vi "NI5112.start scan.vi"(0 "i ref in":refnum<vi>, 3 "ms timeout (100)":i32=100, 5 "error in (no error)":errorcluster) -> (14 "i ref out":refnum<vi>, 17 "timed out":bool, 19 "error out":errorcluster)   [LabVIEW 2014, in "NI5112.lvlib"]
uses:
  NI5112.lvlib
  <instrlib>/niScope/Controls/niScope trigger source.ctl
  <instrlib>/niScope/Controls/niScope trigger slope.ctl
  <instrlib>/niScope/Controls/niScope trigger coupling.ctl
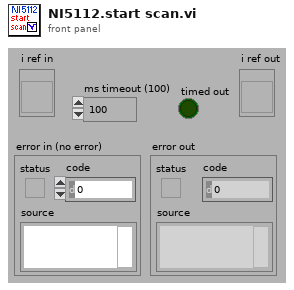
[diagram p1: front panel]
types:
  T1 = typedef "niScope trigger coupling.ctl" = u16
  T2 = typedef "niScope trigger slope.ctl" = i32
  T3 = typedef "niScope trigger source.ctl" = string
  T4 = typedef "NI5112.lvlib/NI5112.i attribute.ctl" = cluster{"HWChannel":string, "instrument handle":refnum<k15>, "BinWidth":dbl, "vertical offset":dbl, "vertical range":dbl, "DataBPR":i32, "5112BPR":i32, "FullSpeed":bool, "discrLevel":dbl, "DoDiscr":bool, "VerCoupling":string}
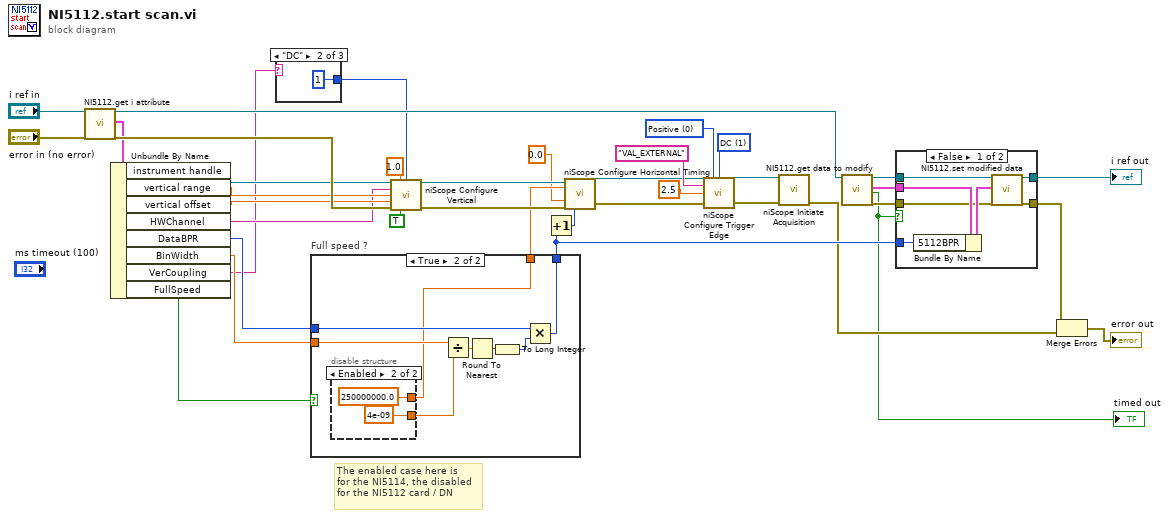
[diagram p0: block diagram]
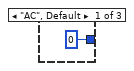
[diagram p2: hidden frame]
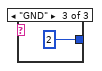
[diagram p3: hidden frame]
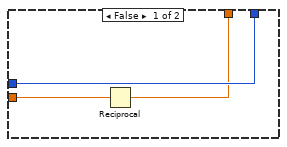
[diagram p4: hidden frame]
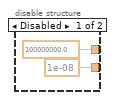
[diagram p5: hidden frame]
diagram:
  w33 = T1 1 items=["AC"=0, "DC"=1, "HF Reject"=3, "LF Reject"=4, "AC Plus HF Reject"=1001] ("trigger coupling")
  w34 = T2 0 items=["Positive", "Negative"] ("trigger slope")
  # "The enabled case here is\nfor the NI5114, the disabled\nfor the NI5112 card / DN"
  n1 = call "NI5112.get i attribute.vi"("i ref in"="i ref in", "error in (no error)"="error in (no error)") -> ("i ref out"=w15:refnum<vi>, "i attribute"=w37:T4, "error out"=w38:errorcluster)  [unwired: 15 in]
  n2 = Unbundle By Name(w37) -> ("instrument handle"=w32:refnum<k15>, "vertical range"=w30:dbl, "vertical offset"=w29:dbl, "HWChannel"=w28:string, "DataBPR"=w19:i32, "BinWidth"=w20:dbl, "VerCoupling"=w2:string, "FullSpeed"=w3:bool)
  n3 = case shown="\"DC\"" w2 {
    tunnel: [0 1 2] -> w1
    frame "AC", Default {
    }
    frame "DC" {
    }
    frame "GND" {
    }
  }
  n4 = case "Full speed ?" shown="True" w3 {
    tunnel: w20 -> [w43 w51]
    tunnel: w19 -> [w44 w48]
    tunnel: [w44 w46] -> w12
    tunnel: [w42 w45] -> w7
    frame False {
      n5 = Reciprocal(x=w43) -> (1/x=w42:dbl)
    }
    frame True {
      n6 = disable-structure shown="Enabled" {
        disable-tunnel: [1e-08 ("min sample rate") 4e-09 ("min sample rate")] -> w52
        disable-tunnel: [100000000.0 ("min sample rate") 250000000.0 ("min sample rate")] -> w45
        frame Disabled {
        }
        frame Enabled {
        }
      }
      n7 = Divide(x=w51, y=w52) -> (x/y=w50:dbl)
      n8 = Round To Nearest(number=w50) -> (nearest integer value=w49:dbl)
      n9 = To Long Integer(number=w49) -> (32bit integer=w47:i32)
      n10 = Multiply(x=w48, y=w47) -> (x*y=w46:i32)
    }
  }
  n11 = call <instrlib>:"niScope Configure Vertical.vi"("instrument handle"=w32, "probe attenuation"=1.0, "vertical coupling"=w1, "channels"=w28, "vertical range"=w30, "vertical offset"=w29, "error in"=w38, "channel enabled"=TRUE) -> ("instrument handle out"=w25:refnum<k15>, "error out"=w26:errorcluster)  [unwired: 6 in]
  n12 = Increment(x=w12) -> (x+1=w18:i32)
  n13 = call <instrlib>:"niScope Configure Horizontal Timing.vi"("instrument handle"=w25, "min sample rate"=w7, "reference position"=0.0, "error in"=w26, "min record length"=w18) -> ("instrument handle out"=w23:refnum<k15>, "error out"=w24:errorcluster)  [unwired: 9 in]
  n14 = call <instrlib>:"niScope Configure Trigger Edge.vi"("instrument handle"=w23, "trigger slope"=w34, "trigger coupling"=w33, "trigger source"=T3 "VAL_EXTERNAL", "trigger level"=2.5, "error in"=w24) -> ("instrument handle out"=w22:refnum<k15>, "error out"=w21:errorcluster)  [unwired: 8 in]
  n15 = call <instrlib>:"niScope Initiate Acquisition.vi"("instrument handle"=w22, "error in"=w21) -> ("error out"=w10:errorcluster)  [unwired: 12 in, 1 out]
  n16 = call "NI5112.get data to modify.vi"("i ref in"=w15) -> ("i ref out"=w14:refnum<vi>, "i attribute"=w17:T4, "timed out"=w8:bool, "error out"=w16:errorcluster)  [unwired: 15 in]
  "timed out" <- w8
  n17 = case shown="False" w8 {
    tunnel: w17 -> [w63 _]
    tunnel: w16 -> [w61 w65]
    tunnel: [w60 w65] -> w11
    tunnel: w14 -> [w59 w64]
    tunnel: [w58 w64] -> w13
    tunnel: w12 -> [w57 _]
    frame False {
      n18 = Bundle By Name(cluster=w63, "5112BPR"=w57) -> (w62:T4)
      n19 = call "NI5112.set modified data.vi"("i ref in"=w59, "i attribute"=w62, "error in (no error)"=w61) -> ("i ref out"=w58:refnum<vi>, "error out"=w60:errorcluster)  [unwired: 15 in]
    }
    frame True {
    }
  }
  "i ref out" <- w13
  n20 = Merge Errors(w11, w10) -> (→"error out":errorcluster)
